vi "storeADCMixedToArray-wang-test2test2.vi"(0 "String":string) -> ()   [LabVIEW 2014]
panel:
  out "initialized array 2":i32[][](array[numeric])
  out "initialized array":i32[][](array[numeric])
  out "Waveform":waveform(dbl)
  out "Numeric 2":i32
  out "Numeric":i32
  out "TotalTrigger":i32
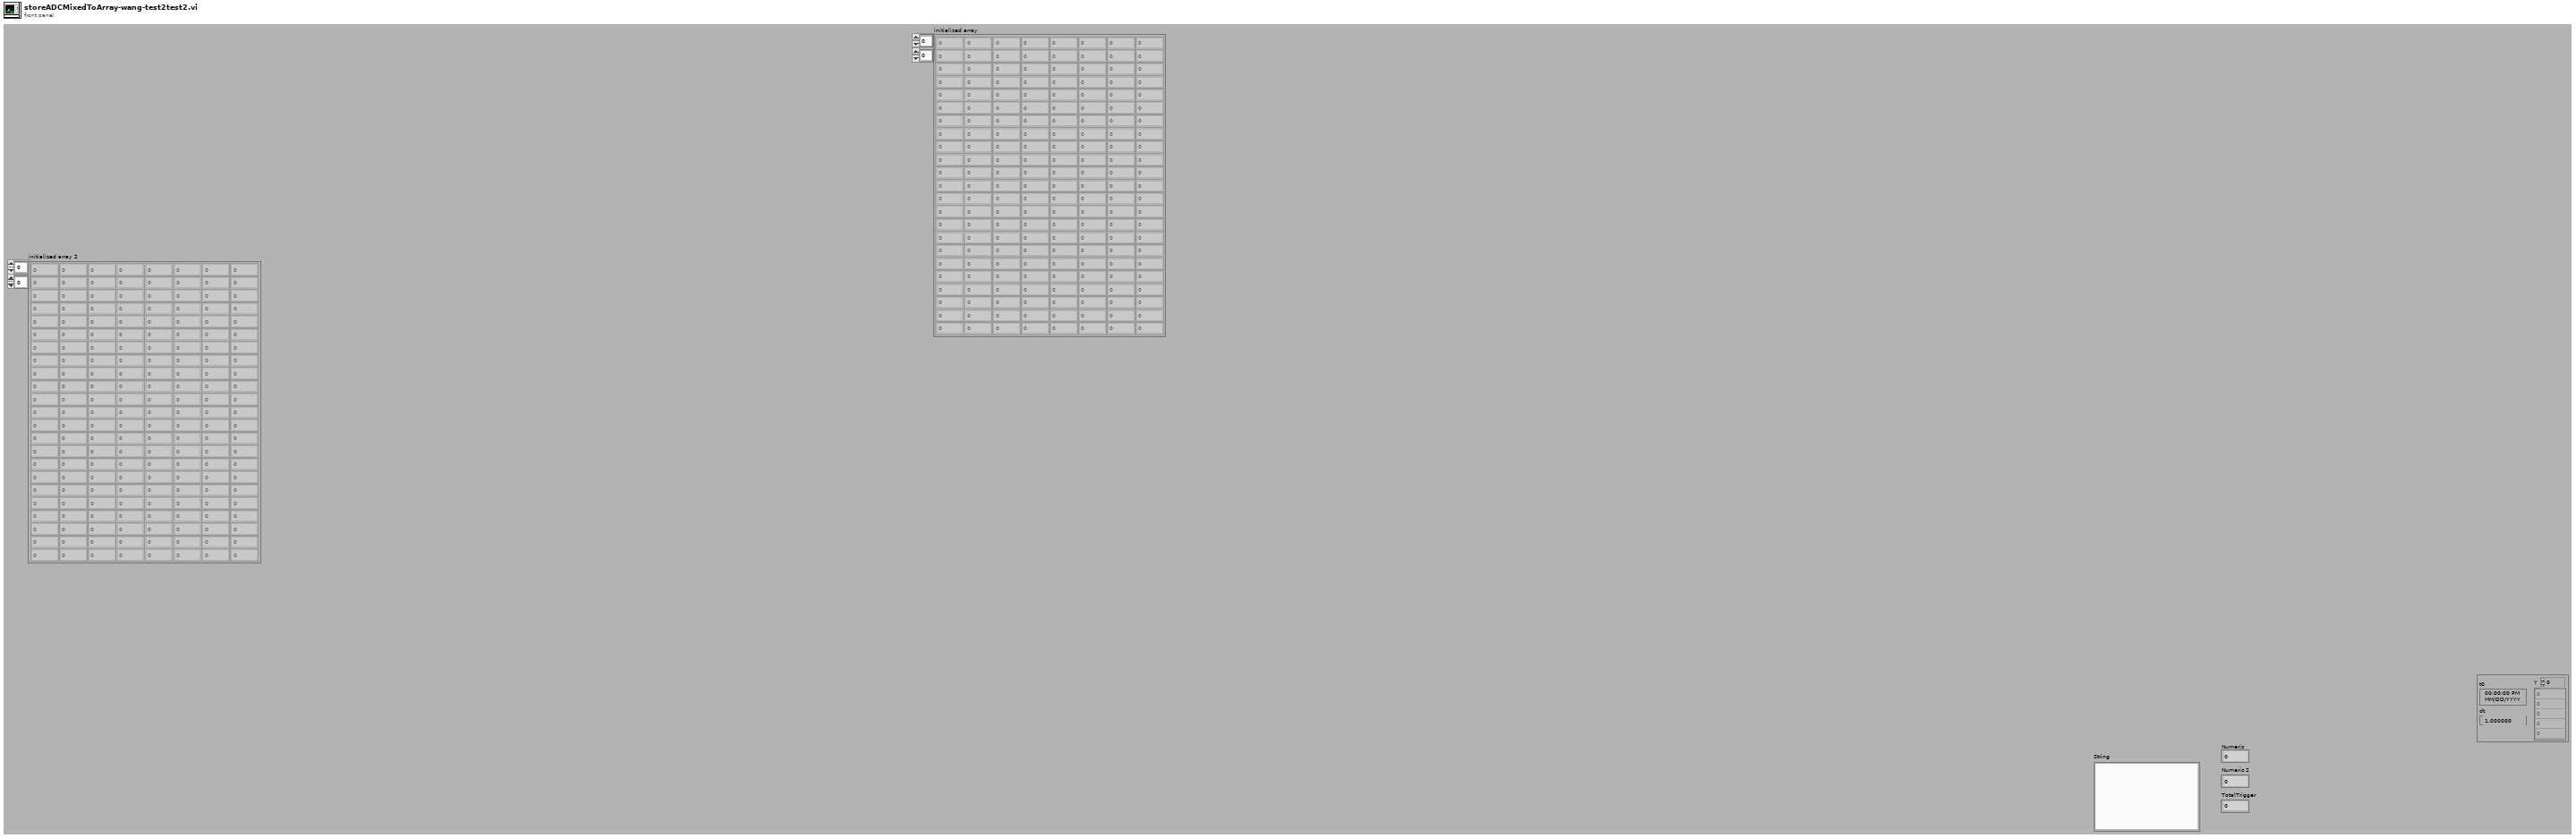
[diagram p1: front panel]
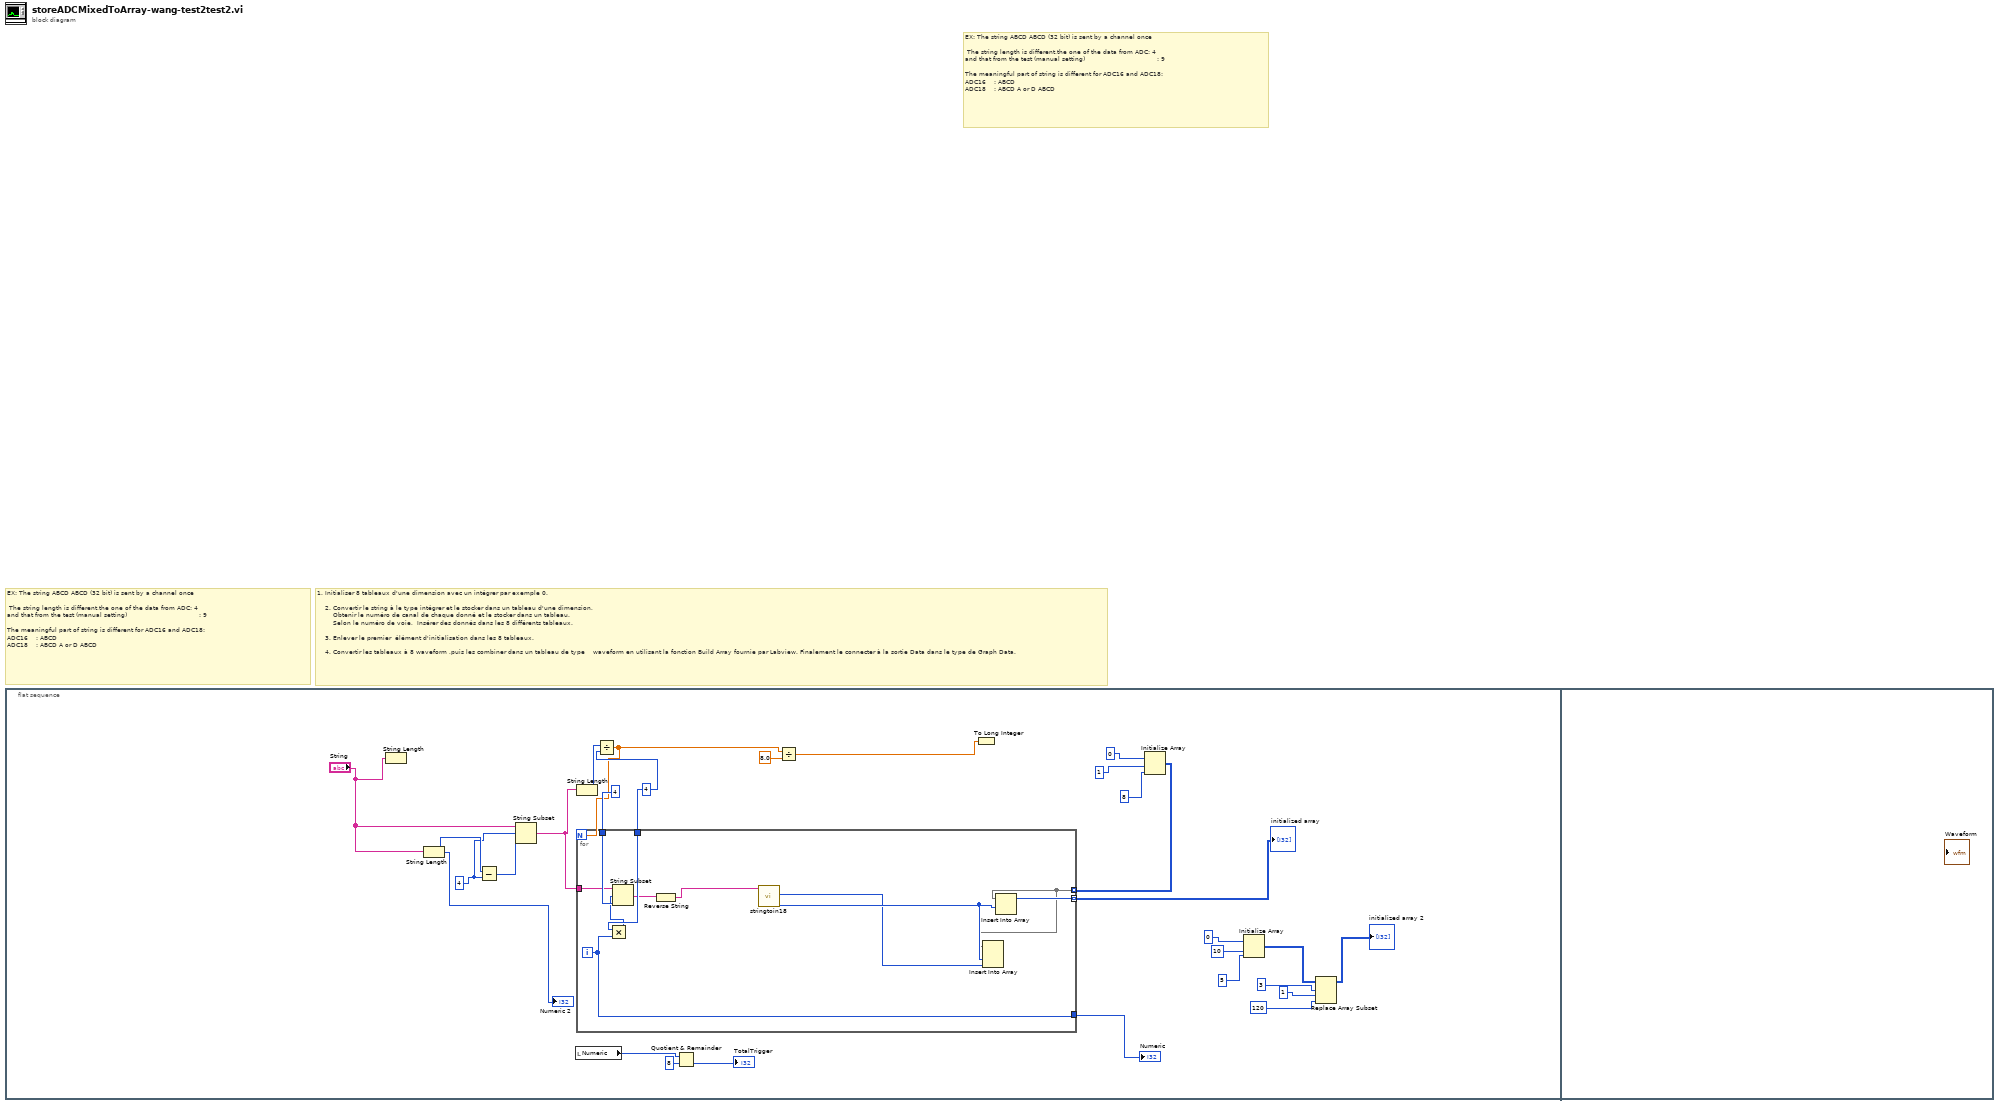
[diagram p0: block diagram]
diagram:
  # "1. Initialiser 8 tableaux d'une dimension avec un intégrer par exemple 0.\n\n    2.\tConvertir le string à le type intégrer et le stocker dans un tableau d'une dimension,\n        Obtenir le numéro de canal de chaque donné et le stocker dans un tableau.  \n        Selon le numéro de voie,  Insérer des donnés dans les 8 différents tableaux.\n\n    3. Enlever le premier  élément d'initialisation dans les 8 tableaux.\n\n    4. Convertir les tableaux à 8 waveform ,puis les combiner dans un tableau de type    waveform en utilisant la fonction Build Array fournie par Labview. Finalement le connecter à la sortie Data dans le type de Graph Data."
  # "EX: The string ABCD ABCD (32 bit) is sent by a channel once                \n\n The string length is different,the one of the data from ADC: 4\nand that from the test (manual setting)                                    : 9\n\nThe meaningful part of string is different for ADC16 and ADC18:\nADC16    : ABCD                          \nADC18    : ABCD A or D ABCD"
  # "EX: The string ABCD ABCD (32 bit) is sent by a channel once                \n\n The string length is different,the one of the data from ADC: 4\nand that from the test (manual setting)                                    : 9\n\nThe meaningful part of string is different for ADC16 and ADC18:\nADC16    : ABCD                          \nADC18    : ABCD A or D ABCD"
  n1 = flat-sequence {
    frame #0 {
      w22 = 4
      w25 = 4
      n2 = String Length(string="String") -> ()  [unwired: 1 out]
      n3 = String Length(string="String") -> (length=w28:i32)
      "Numeric 2" <- w28
      n4 = Subtract(x=w28, y=w25) -> (x-y=w26:i32)
      n5 = String Subset(string="String", offset (0)=w25, length (rest)=w26) -> (substring=w21:string)
      n6 = local read "Numeric"() -> (w18:i32)
      n7 = String Length(string=w21) -> (length=w23:i32)
      n8 = Divide(x=w23, y=w22) -> (x/y=w14:dbl)
      n9 = Quotient & Remainder(x=w18, y=8) -> (floor(x/y)=→"TotalTrigger":i32)  [unwired: 1 out]
      n10 = Divide(x=w14, y=8.0) -> (x/y=w10:dbl)
      n11 = To Long Integer(number=w10) -> ()  [unwired: 1 out]
      n12 = Initialize Array(0, 1, 8) -> (w9:i32[][])
      n13 = for {
        N: w14 -> [_]
        tunnel: 4 -> [w39]
        tunnel: w22 -> [w38]
        tunnel: [w34] -> w27
        tunnel: w21 -> [w35]
        tunnel: w9 -> [w29] mode=indexing
        tunnel: [w32] -> w11 mode=indexing
        i -> [w34]
        n14 = Multiply(x=w38, y=w34) -> (x*y=w37:i32)
        n15 = String Subset(string=w35, offset (0)=w37, length (rest)=w39) -> (substring=w36:string)
        n16 = Reverse String(1:w36) -> (0:w33:string)
        n17 = call "stringtoin18.vi"("input_string"=w33) -> ("channel"=w31:u8, "outputComplemented_int"=w30:i32)  [unwired: 7 in, 2 out]
        n18 = Insert Into Array(array=w29, index (col)=w31, new element=w30) -> ()  [unwired: 1 in, 1 out]
        n19 = Insert Into Array(array=w29, index=w31) -> (w32:i32[])  [unwired: 1 in]
      }
      "Numeric" <- w27
      "initialized array" <- w11
      n20 = Initialize Array(0, 10, 5) -> (w4:i32[][])
      n21 = Replace Array Subset(array=w4, new element=120, index (row)=3, index (col)=1) -> (→"initialized array 2":i32[][])
    }
    frame #1 {
    }
  }
